vi "Grab and Scalable Format.vi"() -> ()   [LabVIEW 2011]
doc: "The Grab and Scalable Format VI acquires images continuously and displays the images in an image control using high-level acquisition VIs. A grab is appropriate for high-speed applications in which you need to process only one image at a time. This example requires a GigE Vision camera or a FireWire camera that supports Partial Image Size Format (Format 7)."
uses:
  <vilib>/vision/driver/NI_Vision_Acquisition_Software.lvlib
  resource/objmgr/imaqdx.rc
panel:
  in  "Camera Name":refnum<k21> caption="IMAQdx Session"
  in  "Image Size Parameters":T1={"Offset X"=130, "Offset Y"=175, "Width"=423, "Height"=332, "Packet Size"=2679} {"Packet Size" scale=0.0..4096.0; "Width" scale=0.0..1024.0; "Offset X" scale=0.0..1024.0}
  out "Image":T2(plugin-control)
  out "Frame Rate":dbl(knob) scale=0.0..100.0
  in  "Stop":bool
  # "Overview: Demonstrates how to modify the Partial Image Size Format (Format 7) settings while acquiring images.\nRequirements: Vision Acquisition Software, a GigE Vision camera or a FireWire camera that supports Partial Image Size Format (Format 7).\nInstructions:\n1. Select the Camera Name\n2. Run the VI\n3. Adjust the Image Size Parameters"
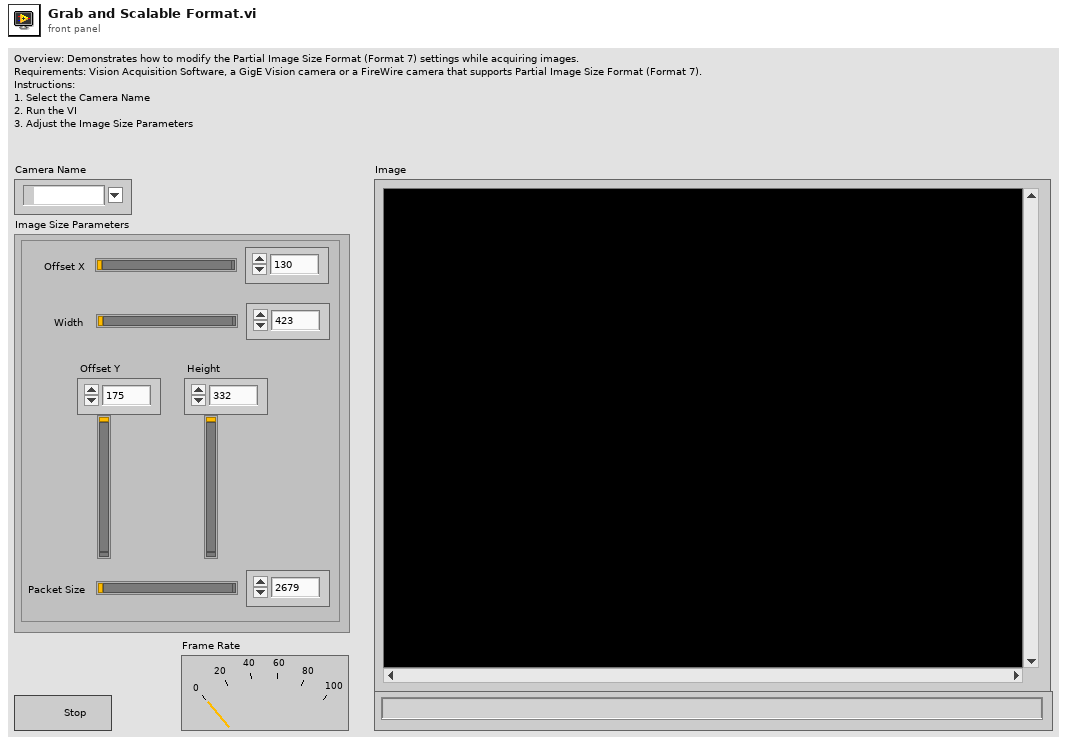
[diagram p1: front panel]
types:
  T1 = cluster{"Offset X":u32, "Offset Y":u32, "Width":u32, "Height":u32, "Packet Size":u32}
  T2 = typedef "IMAQ Image.ctl" = refnum<image>
  T3 = typedef "IMAQdx.ctl" = refnum<k21>
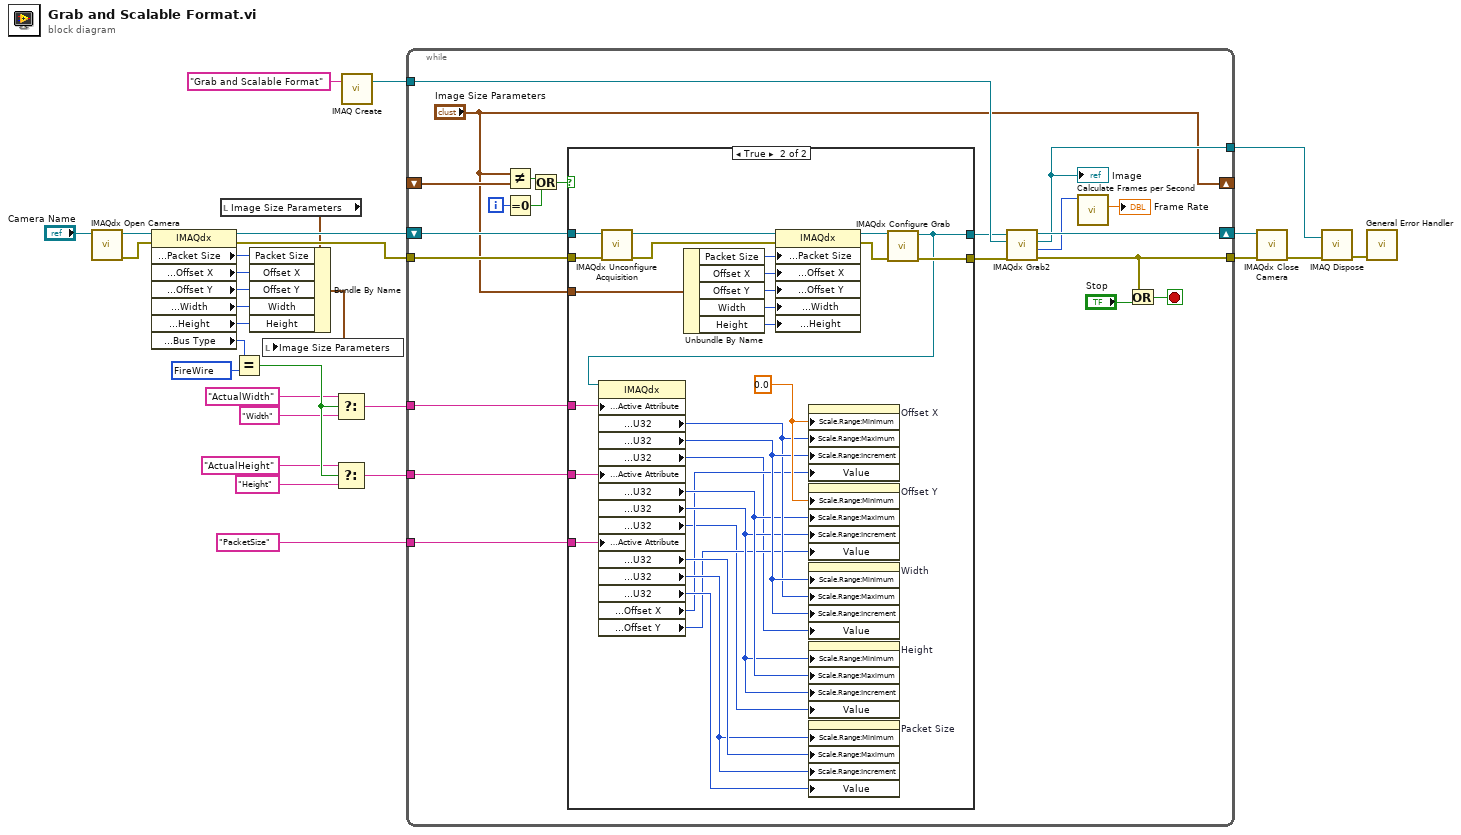
[diagram p0: block diagram]
diagram:
  w14 = u32 825440564 items=["FireWire"=825440564, "Ethernet"=1768977972] ("BusType")
  n1 = call <vilib>:"IMAQdx Open Camera.vi"("Session In"="Camera Name") -> ("error out"=w24:errorcluster, "Session Out"=w25:T3)  [unwired: 2 in, 7 out]
  n2 = property class="IMAQdx"(reference=w25, error in=w24) -> (reference out=w18:T3, error out=w17:errorcluster, "Acquisition Attributes:Packet Size"=w23:u32, "Acquisition Attributes:Offset X"=w22:u32, "Acquisition Attributes:Offset Y"=w21:u32, "Acquisition Attributes:Width"=w20:u32, "Acquisition Attributes:Height"=w19:u32, "Camera Information:Bus Type"=w13:u32)
  n3 = local read "Image Size Parameters"() -> (w15:T1)
  n4 = Equal?(x=w13, y=w14) -> (x = y?=w12:bool)
  n5 = Bundle By Name(cluster=w15, "Packet Size"=w23, "Offset X"=w22, "Offset Y"=w21, "Width"=w20, "Height"=w19) -> (w16:T1)
  n6 = local write "Image Size Parameters"(w16) -> ()
  n7 = Select(t="ActualWidth" ("ActiveAttribute"), s=w12, f="Width" ("ActiveAttribute")) -> (s? t:f=w10:string)
  n8 = Select(t="ActualHeight" ("ActiveAttribute"), s=w12, f="Height" ("ActiveAttribute")) -> (s? t:f=w8:string)
  n9 = call "IMAQ Create"("Image Name"="Grab and Scalable Format") -> ("New Image"=w29:T2)  [unwired: 3 in, 2 out]
  n10 = while {
    tunnel: [w32] -> w27
    tunnel: w29 -> [w48]
    shift-right: ["Image Size Parameters"] -> _
    shift-left: _ -> [w41]
    tunnel: w17 -> [w43]
    shift-right: [w47] -> w28
    shift-left: w18 -> [w44]
    tunnel: w10 -> [w37]
    tunnel: w8 -> [w36]
    tunnel: "PacketSize" ("ActiveAttribute") -> [w35]
    tunnel: [w31] -> w3
    i -> [w42]
    stop <- w50 stop-if-true
    n11 = Not Equal?(x="Image Size Parameters", y=w41) -> (x != y?=w33:bool)
    n12 = Equal To 0?(x=w42) -> (x = 0?=w40:bool)
    n13 = Or(x=w33, y=w40) -> (x .or. y?=w39:bool)
    n14 = case shown="True" w39 {
      tunnel: [w51 w81] -> w46
      tunnel: [w52 w71] -> w45
      tunnel: w44 -> [w52 w80]
      tunnel: w43 -> [w51 w78]
      tunnel: w37 -> [_ w56]
      tunnel: w36 -> [_ w55]
      tunnel: w35 -> [_ w54]
      tunnel: "Image Size Parameters" -> [_ w53]
      frame False {
      }
      frame True {
        w75 = 0.0 ("Scale.Range:Minimum")
        n15 = call <vilib>:"IMAQdx Unconfigure Acquisition.vi"("error in"=w78, "Session In"=w80) -> ("error out"=w76:errorcluster, "Session Out"=w79:T3)  [unwired: 8 out]
        n16 = Unbundle By Name(w53) -> ("Packet Size"=w69:u32, "Offset X"=w68:u32, "Offset Y"=w70:u32, "Width"=w67:u32, "Height"=w66:u32)
        n17 = property class="IMAQdx"(reference=w79, error in=w76, "Acquisition Attributes:Packet Size"=w69, "Acquisition Attributes:Offset X"=w68, "Acquisition Attributes:Offset Y"=w70, "Acquisition Attributes:Width"=w67, "Acquisition Attributes:Height"=w66) -> (reference out=w77:T3, error out=w74:errorcluster)
        n18 = call <vilib>:"IMAQdx Configure Grab.vi"("error in"=w74, "Session In"=w77) -> ("error out"=w81:errorcluster, "Session Out"=w71:T3)  [unwired: 1 in, 7 out]
        n19 = property class="IMAQdx"(reference=w71, "Camera Attributes:Active Attribute"=w56, "Camera Attributes:Active Attribute"=w55, "Camera Attributes:Active Attribute"=w54) -> ("Camera Attributes:Maximum:U32"=w72:u32, "Camera Attributes:Minimum:U32"=w73:u32, "Camera Attributes:Value:U32"=w58:u32, "Camera Attributes:Maximum:U32"=w65:u32, "Camera Attributes:Minimum:U32"=w64:u32, "Camera Attributes:Value:U32"=w57:u32, "Camera Attributes:Maximum:U32"=w63:u32, "Camera Attributes:Minimum:U32"=w62:u32, "Camera Attributes:Value:U32"=w61:u32, "Acquisition Attributes:Offset X"=w60:u32, "Acquisition Attributes:Offset Y"=w59:u32)  [unwired: 1 in, 2 out]
        n20 = property on="Offset X" class="Slide (strict)"("Scale.Range:Minimum"=w75, "Scale.Range:Maximum"=w72, "Scale.Range:Increment"=w73, "Value"=w60) -> ()  [unwired: 2 in, 2 out]
        n21 = property on="Offset Y" class="Slide (strict)"("Scale.Range:Minimum"=w75, "Scale.Range:Maximum"=w65, "Scale.Range:Increment"=w64, "Value"=w59) -> ()  [unwired: 2 in, 2 out]
        n22 = property on="Width" class="Slide (strict)"("Scale.Range:Minimum"=w73, "Scale.Range:Maximum"=w72, "Scale.Range:Increment"=w73, "Value"=w58) -> ()  [unwired: 2 in, 2 out]
        n23 = property on="Height" class="Slide (strict)"("Scale.Range:Minimum"=w64, "Scale.Range:Maximum"=w65, "Scale.Range:Increment"=w64, "Value"=w57) -> ()  [unwired: 2 in, 2 out]
        n24 = property on="Packet Size" class="Slide (strict)"("Scale.Range:Minimum"=w62, "Scale.Range:Maximum"=w63, "Scale.Range:Increment"=w62, "Value"=w61) -> ()  [unwired: 2 in, 2 out]
      }
    }
    n25 = call <vilib>:"IMAQdx Grab2.vi"("error in"=w46, "Image In"=w48, "Session In"=w45) -> ("error out"=w32:errorcluster, "Buffer Number Out"=w34:u32, "Image Out"=w31:T2, "Session Out"=w47:T3)  [unwired: 5 in]
    "Image" <- w31
    n26 = call <vilib>:"Calculate Frames per Second.vi"("Buffer Number"=w34) -> ("Processed Frames/s"=→"Frame Rate":dbl)  [unwired: 8 in, 2 out]
    n27 = Or(x=w32, y="Stop") -> (x .or. y?=w50:bool)
  }
  n28 = call <vilib>:"IMAQdx Close Camera.vi"("error in"=w27, "Session In"=w28) -> ("error out"=w2:errorcluster)  [unwired: 9 out]
  n29 = call "IMAQ Dispose"("Image"=w3, "error in (no error)"=w2) -> ("error out"=w1:errorcluster)  [unwired: 4 in]
  n30 = call <vilib>:"General Error Handler.vi"("error in (no error)"=w1) -> ()  [unwired: 1 in, 14 out]
